vi "test.vi"() -> ()   [LabVIEW 2014]
panel:
  out "test point val (qu step)":dbl
  out "Raw Val":u16 format="%.0x"
  out "Test Point Val (V)":dbl
  in  "Address (0x50)":u16=80 max=1023 format="%.0x"
  out "error out":errorcluster
  out "Pullup?":bool
  out "Aardvark Power Enable":bool
  out "Bit Rate":i16
  in  "error in (no error)":errorcluster
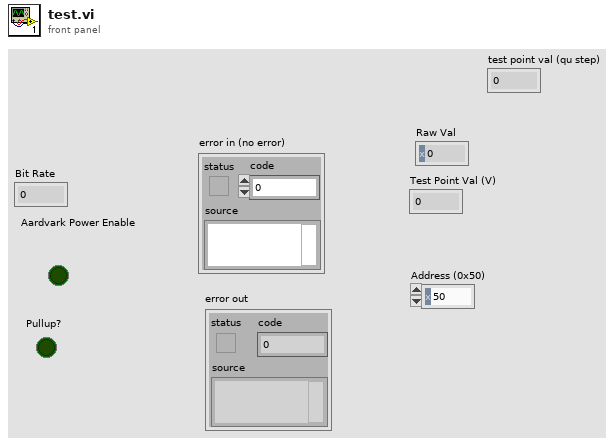
[diagram p1: front panel]
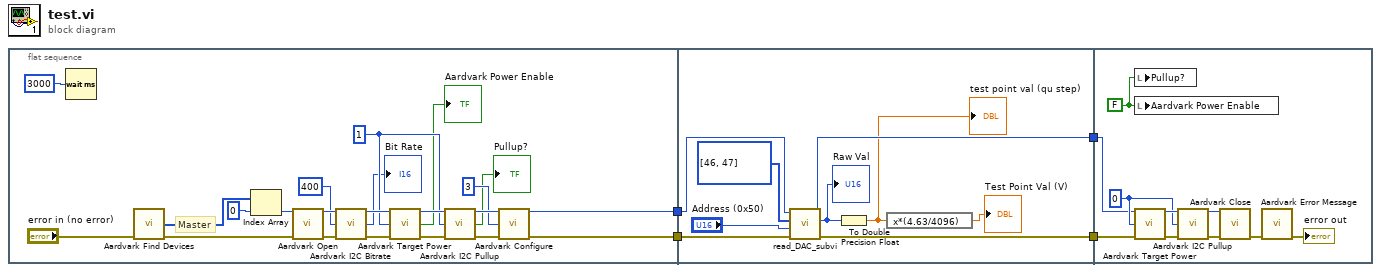
[diagram p0: block diagram]
diagram:
  n1 = flat-sequence {
    tunnel: [w7] -> w4
    tunnel: [w6] -> w2
    tunnel: w4 -> [w32]
    tunnel: [w28] -> w3
    tunnel: w2 -> [w34]
    tunnel: [w33] -> w1
    tunnel: w3 -> [w39]
    tunnel: w1 -> [w38]
    frame #0 {
      w12 = 1
      # "Master"
      n2 = Wait (ms)(milliseconds to wait=3000) -> ()  [unwired: 1 out]
      n3 = call <instrlib>:"Aardvark Find Devices.vi"("error in (no error)"="error in (no error)") -> ("Ports"=w25:u16[], "error out"=w24:errorcluster)  [unwired: 12 in, 1 out]
      n4 = Index Array(array=w25, index=0) -> (element=w23:u16)
      n5 = call <instrlib>:"Aardvark Open.vi"("Port Number (0)"=w23, "error in (no error)"=w24) -> ("Aardvark Handle"=w21:i32, "error out"=w17:errorcluster)  [unwired: 12 in]
      n6 = call <instrlib>:"Aardvark I2C Bitrate.vi"("Aardvark Handle"=w21, "Requested Bitrate kHz (100)"=400, "error in (no error)"=w17) -> ("dup Aardvark Handle"=w20:i32, "Actual Bitrate kHz"=→"Bit Rate":i32, "error out"=w16:errorcluster)  [unwired: 10 in]
      n7 = call <instrlib>:"Aardvark Target Power.vi"("Aardvark Handle"=w20, "Requested Configuration (2: Query)"=w12, "error in (no error)"=w16) -> ("dup Aardvark Handle"=w19:i32, "Target Power Enabled?"=→"Aardvark Power Enable":bool, "error out"=w15:errorcluster)  [unwired: 10 in]
      n8 = call <instrlib>:"Aardvark I2C Pullup.vi"("Aardvark Handle"=w19, "Requested Configuration (query)"=w12, "error in (no error)"=w15) -> ("dup Aardvark Handle"=w18:i32, "Pullups Enabled?"=→"Pullup?":bool, "error out"=w14:errorcluster)  [unwired: 10 in]
      n9 = call <instrlib>:"Aardvark Configure.vi"("Aardvark Handle"=w18, "Requested Configuration (0x80: Query)"=3, "error in (no error)"=w14) -> ("dup Aardvark Handle"=w7:i32, "error out"=w6:errorcluster)  [unwired: 10 in, 1 out]
    }
    frame #1 {
      n10 = call "read_DAC_subvi.vi"("error in (no error)"=w34, "Address (0x50)"="Address (0x50)", "DAC_ADD"=u8[] [46, 47], "Aardvark Handle"=w32) -> ("error out"=w33:errorcluster, "DAC Val"=w29:u16, "Dup Aardvark Handle"=w28:i32)  [unwired: 3 in]
      "Raw Val" <- w29
      n11 = To Double Precision Float(number=w29) -> (double precision float=w27:dbl)
      "test point val (qu step)" <- w27
      n12 = expression code="x*(4.63/4096)"(w27) -> (→"Test Point Val (V)":dbl)
    }
    frame #2 {
      w37 = FALSE
      w40 = 0
      n13 = local write "Pullup?"(w37) -> ()
      n14 = local write "Aardvark Power Enable"(w37) -> ()
      n15 = call <instrlib>:"Aardvark Target Power.vi"("Aardvark Handle"=w39, "Requested Configuration (2: Query)"=w40, "error in (no error)"=w38) -> ("dup Aardvark Handle"=w43:i32, "error out"=w41:errorcluster)  [unwired: 10 in, 1 out]
      n16 = call <instrlib>:"Aardvark I2C Pullup.vi"("Aardvark Handle"=w43, "Requested Configuration (query)"=w40, "error in (no error)"=w41) -> ("dup Aardvark Handle"=w42:i32, "error out"=w36:errorcluster)  [unwired: 10 in, 1 out]
      n17 = call <instrlib>:"Aardvark Close.vi"("Aardvark Handle"=w42, "error in (no error)"=w36) -> ("error out"=w44:errorcluster)  [unwired: 13 in]
      n18 = call <instrlib>:"Aardvark Error Message.vi"("error in (no error)"=w44) -> ("error out"=→"error out":errorcluster)  [unwired: 10 in, 4 out]
    }
  }
